vi "PresetExecutionDataCluster.vi"() -> (0 "Preset Manager Cluster":T1)   [LabVIEW 2020]
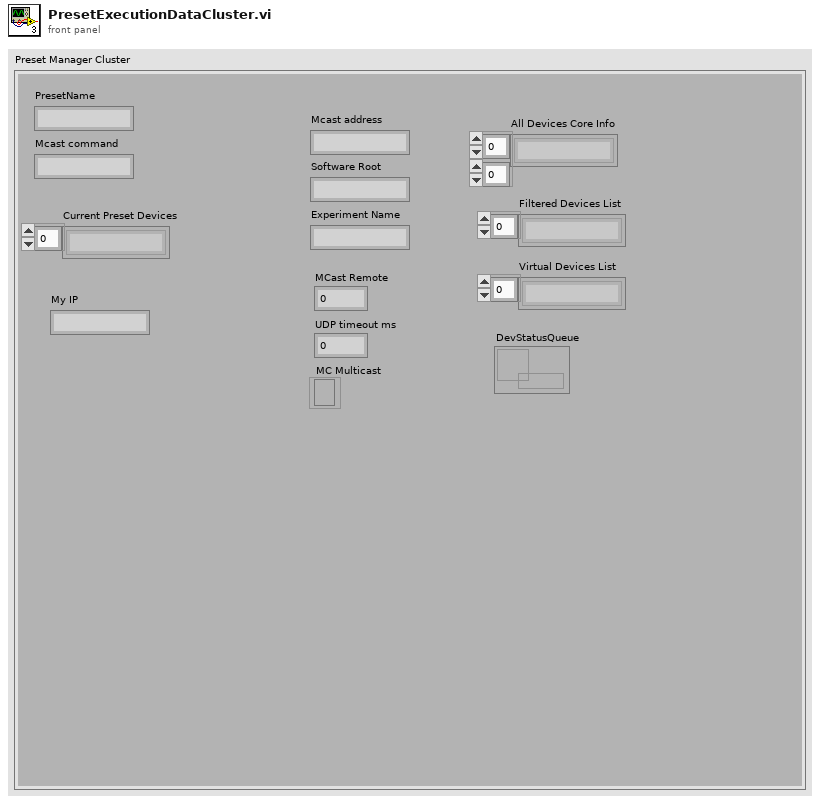
[diagram p1: front panel]
types:
  T1 = cluster{"PresetName":string, "Mcast command":string, "Current Preset Devices":string[], "My IP":string, "Mcast address":string, "Software Root":string, "Experiment Name":string, "MCast Remote":u16, "UDP timeout ms":i32, "MC Multicast":refnum<k16>, "All Devices Core Info":string[][], "Filtered Devices List":string[], "Virtual Devices List":string[], "DevStatusQueue":refnum<queue>}
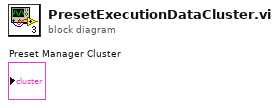
[diagram p0: block diagram]
diagram:
